vi "Z equivalent (SubVI) RT.vi"(0 "Actual SOC( / )":dbl) -> (4 "Rseries(soc)":dbl, 6 "R transient_S(soc)":dbl, 8 "C transient_S(soc)":dbl, 10 "R transient_L(soc)":dbl, 15 "C transient_L(soc)":dbl)   [LabVIEW 2016]
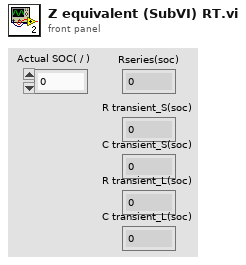
[diagram p1: front panel]
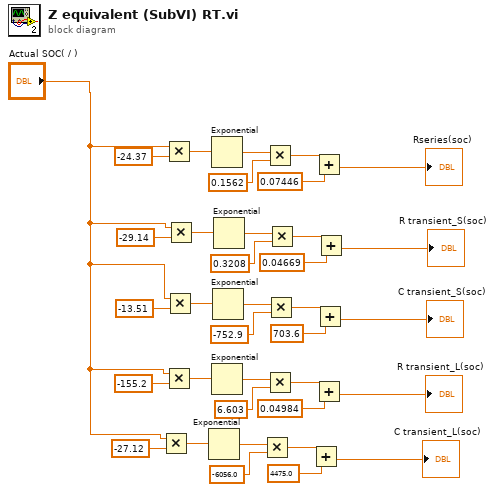
[diagram p0: block diagram]
diagram:
  n1 = Multiply(x="Actual SOC( / )", y=-27.12) -> (x*y=w7:dbl)
  n2 = Multiply(x="Actual SOC( / )", y=-24.37) -> (x*y=w35:dbl)
  n3 = Multiply(x="Actual SOC( / )", y=-155.2) -> (x*y=w14:dbl)
  n4 = Multiply(x="Actual SOC( / )", y=-13.51) -> (x*y=w21:dbl)
  n5 = Multiply(x="Actual SOC( / )", y=-29.14) -> (x*y=w28:dbl)
  n6 = Exponential(1:w7) -> (0:w6:dbl)
  n7 = Exponential(1:w35) -> (0:w34:dbl)
  n8 = Exponential(1:w14) -> (0:w13:dbl)
  n9 = Exponential(1:w21) -> (0:w20:dbl)
  n10 = Exponential(1:w28) -> (0:w27:dbl)
  n11 = Multiply(x=w6, y=-6056.0) -> (x*y=w4:dbl)
  n12 = Multiply(x=w34, y=0.1562) -> (x*y=w32:dbl)
  n13 = Multiply(x=w13, y=6.603) -> (x*y=w11:dbl)
  n14 = Multiply(x=w20, y=-752.9) -> (x*y=w18:dbl)
  n15 = Multiply(x=w27, y=0.3208) -> (x*y=w25:dbl)
  n16 = Add(x=w4, y=4475.0) -> (x+y=→"C transient_L(soc)":dbl)
  n17 = Add(x=w32, y=0.07446) -> (x+y=→"Rseries(soc)":dbl)
  n18 = Add(x=w11, y=0.04984) -> (x+y=→"R transient_L(soc)":dbl)
  n19 = Add(x=w18, y=703.6) -> (x+y=→"C transient_S(soc)":dbl)
  n20 = Add(x=w25, y=0.04669) -> (x+y=→"R transient_S(soc)":dbl)
